vi "Get configuration chain.vi"(8 "error in (no error)":errorcluster, 11 "ExampleClassA in":refnum<class "ExampleClassA.lvclass">) -> (0 "error out":errorcluster, 1 "class name":string[](array[string]), 2 "configuration chain":variant[](array[variant]), 3 "ExampleClassA out":refnum<class "ExampleClassA.lvclass">)   [LabVIEW 2012, in "ExampleClassA.lvclass"]
doc: "Returns an array of variants containing the configuration clusters of each class in the inheritance chain (lowest child class first), together with an array of all class names in the inheritance chain.\n\nFor classes without configuration cluster, the configuration chain contains empty variants."
uses:
  ExampleClassA.lvclass
  <vilib>/Distrio/Murmex/Murmex/Murmex.lvclass
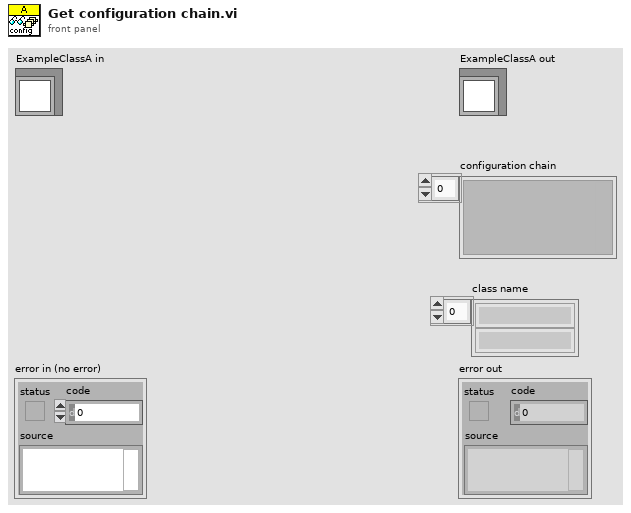
[diagram p1: front panel]
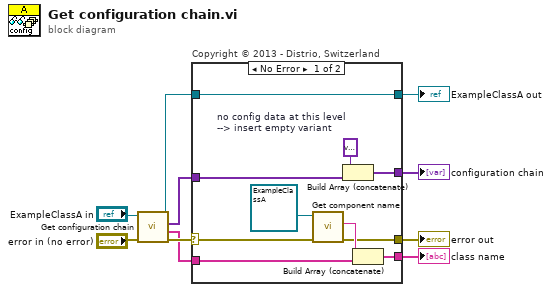
[diagram p0: block diagram]
diagram:
  n1 = call-parent "Get configuration chain.vi"("error in (no error)"="error in (no error)", "MurmexBase in"="ExampleClassA in") -> ("error out"=w10:errorcluster, "class name"=w7:string[], "configuration chain"=w8:variant[], "MurmexBase out"=w9:refnum<class "ExampleClassA.lvclass">)  [unwired: 6 in]
  n2 = case "Copyright © 2013 - Distrio, Switzerland" shown="No Error" w10 {
    selector: w10 -> [w20 w22]
    tunnel: [w13 w22] -> w3
    tunnel: [w18 _] -> w4
    tunnel: [w17 _] -> w6
    tunnel: [w11 w21] -> w5
    tunnel: w9 -> [w11 w21]
    tunnel: w8 -> [w15 _]
    tunnel: w7 -> [w16 _]
    frame No Error {
      w14 = variant  # no config data at this level --> insert empty variant
      n3 = call <vilib>:"Get component name.vi"("error in (no error)"=w20, "Murmex in"=refnum<class "ExampleClassA.lvclass"> refnum ("ExampleClassA")) -> ("error out"=w13:errorcluster, "component name"=w19:string)  [unwired: 7 in, 1 out]
      n4 = Build Array (concatenate)(w14, w15) -> (w17:variant[])
      n5 = Build Array (concatenate)(w19, w16) -> (w18:string[])
    }
    frame Error {
    }
  }
  "error out" <- w3
  "ExampleClassA out" <- w5
  "configuration chain" <- w6
  "class name" <- w4
